vi "Data Directory.vi"(8 "error in (no error)":errorcluster, 10 "Subdirectory":path, 11 "Create if doesn't exist? (F)":bool) -> (0 "error out":errorcluster, 3 "Data directory":path)   [LabVIEW 2020]
uses:
  <vilib>/Utility/sysdir.llb/System Directory Type.ctl
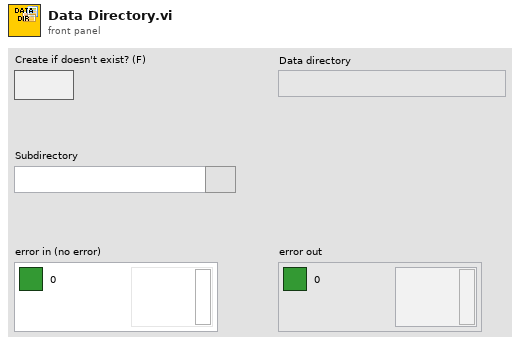
[diagram p1: front panel]
types:
  T1 = typedef "System Directory Type.ctl" = i32
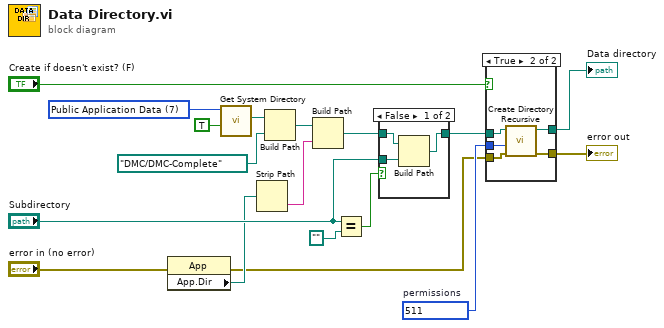
[diagram p0: block diagram]
diagram:
  w7 = i16 511  # permissions
  w17 = T1 7 items=["User Home"=0, "User Desktop"=1, "User Documents"=2, "User Application Data"=3, "User Preferences"=4, "User Temporary"=5, "Public Documents"=6, "Public Application Data"=7, "Public Preferences"=8, "Public Cache"=13, "System Core Libraries"=9, "System Installed Libraries"=10, "Application Files"=11, "Boot Volume Root"=12] ("system directory type")
  n1 = property class="App"(error in="error in (no error)") -> (error out=w4:errorcluster, "App.Dir"=w6:path)  [unwired: 1 in, 1 out]
  n2 = call <vilib>:"Get System Directory.vi"("create directory if not found? (F)"=TRUE, "system directory type"=w17) -> ("system directory"=w15:path)  [unwired: 9 in]
  n3 = Strip Path(path=w6) -> (name=w1:string)  [unwired: 1 out]
  n4 = Build Path(base path=w15, name or relative path=path "DMC/DMC-Complete") -> (appended path=w3:path)
  n5 = Build Path(base path=w3, name or relative path=w1) -> (appended path=w2:path)
  n6 = Equal?(x="Subdirectory", y=path "" ("Subdirectory")) -> (x = y?=w10:bool)
  n7 = case shown="False" w10 {
    tunnel: w2 -> [w21 w22]
    tunnel: [w20 w22] -> w9
    tunnel: "Subdirectory" -> [w19 _]
    frame False {
      n8 = Build Path(base path=w21, name or relative path=w19) -> (appended path=w20:path)
    }
    frame True {
    }
  }
  n9 = case shown="True" "Create if doesn't exist? (F)" {
    tunnel: [w24 w29] -> w14
    tunnel: w9 -> [w24 w28]
    tunnel: w4 -> [w23 w27]
    tunnel: [w23 w26] -> w8
    tunnel: w7 -> [_ w25]
    frame False {
    }
    frame True {
      n10 = call <vilib>:"Create Directory Recursive.vi"("error in (no error)"=w27, "permissions"=w25, "directory"=w28) -> ("error out"=w26:errorcluster, "directory copy"=w29:path)  [unwired: 2 in, 1 out]
    }
  }
  "Data directory" <- w14
  "error out" <- w8
